vi "sonarPositionUpdate.vi"(1 "Obstacles":dbl[][](array[numeric]), 2 "Robot Properties In":T1={"Position"=[0.0, 0.0], "Size"=50.0, "Facing"=0.0, "Movement Ratios"=[0.0, -1.0], "Wheel Angle"=0.0}) -> (0 "Robot Properties Out":T1={"Position"=[0.0, 0.0], "Size"=50.0, "Facing"=0.0, "Movement Ratios"=[0.0, -1.0], "Wheel Angle"=0.0})   [LabVIEW 2015]
uses:
  Robot.ctl
  class/SonarSensor.lvclass
  class/Car.lvclass
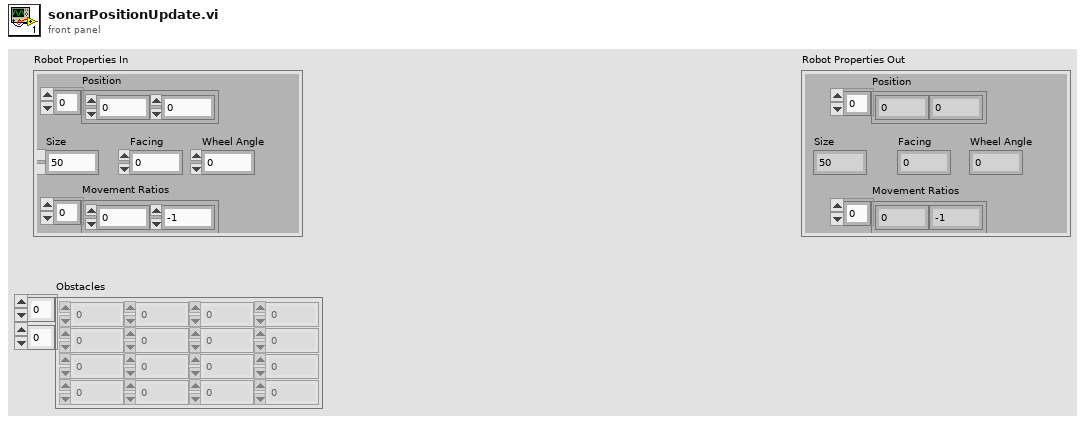
[diagram p1: front panel]
types:
  T1 = typedef "Robot.ctl" = cluster{"Position":dbl[], "Size":dbl, "Facing":dbl, "Movement Ratios":dbl[], "Wheel Angle":dbl}
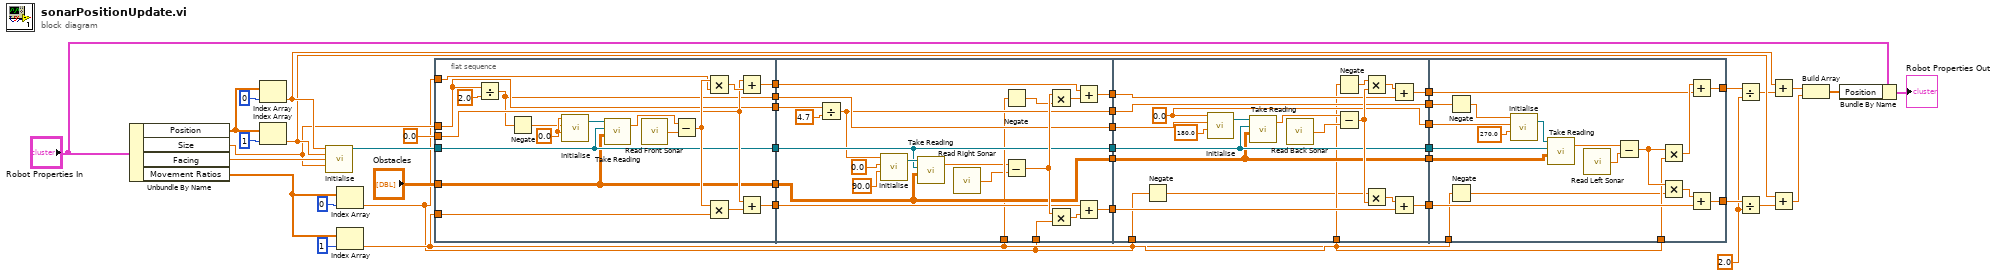
[diagram p0: block diagram]
diagram:
  w2 = 2.0 ("y")
  n1 = Unbundle By Name("Robot Properties In") -> ("Position"=w42:dbl[], "Size"=w24:dbl, "Facing"=w40:dbl, "Movement Ratios"=w37:dbl[])
  n2 = Index Array(array=w42, index=0) -> (element=w28:dbl)
  n3 = Index Array(array=w42, index=1) -> (element=w27:dbl)
  n4 = call "Initialise.vi"("X"=w28, "Y"=w27, "Facing"=w40, "Size"=w24) -> ("Car.lvclass"=w38:refnum<class "Car.lvclass">)  [unwired: 10 in, 1 out]
  n5 = Index Array(array=w37, index=0) -> (element=w6:dbl)
  n6 = Index Array(array=w37, index=1) -> (element=w7:dbl)
  n7 = flat-sequence {
    tunnel: w38 -> [w48]
    tunnel: "Obstacles" -> [w47]
    tunnel: w6 -> [w46]
    tunnel: w7 -> [w45]
    tunnel: 0.0 -> [w52]
    tunnel: [w54] -> w26
    tunnel: [w53] -> w25
    tunnel: w24 -> [w49]
    tunnel: [w49] -> w23
    tunnel: [w48] -> w22
    tunnel: [w47] -> w21
    tunnel: [w44] -> w17
    tunnel: w26 -> [w74]
    tunnel: w25 -> [w73]
    tunnel: w23 -> [w81]
    tunnel: w22 -> [w72]
    tunnel: w21 -> [w71]
    tunnel: [w72] -> w20
    tunnel: [w71] -> w19
    tunnel: [w70] -> w18
    tunnel: w17 -> [w70]
    tunnel: [w69] -> w16
    tunnel: [w68] -> w15
    tunnel: [w67] -> w11
    tunnel: w6 -> [w66]
    tunnel: w7 -> [w64]
    tunnel: w20 -> [w92]
    tunnel: w19 -> [w91]
    tunnel: w18 -> [w100]
    tunnel: w16 -> [w94]
    tunnel: w15 -> [w93]
    tunnel: [w92] -> w14
    tunnel: [w91] -> w13
    tunnel: [w90] -> w12
    tunnel: w11 -> [w89]
    tunnel: [w89] -> w10
    tunnel: [w87] -> w9
    tunnel: [w86] -> w8
    tunnel: w6 -> [w85]
    tunnel: w7 -> [w83]
    tunnel: w14 -> [w120]
    tunnel: w13 -> [w119]
    tunnel: w12 -> [w118]
    tunnel: w10 -> [w116]
    tunnel: w9 -> [w111]
    tunnel: w8 -> [w110]
    tunnel: [w109] -> w3
    tunnel: [w108] -> w4
    tunnel: w7 -> [w107]
    tunnel: w6 -> [w104]
    frame #0 {
      w61 = 0.0
      n8 = Divide(x=w49, y=2.0) -> (x/y=w44:dbl)
      n9 = Negate(x=w44) -> (-x=w50:dbl)
      n10 = call "Initialise.vi"("Facing"=w61, "Y"=w50, "X"=w61) -> ("SonarSensor.lvclass"=w60:refnum<class "SonarSensor.lvclass">)  [unwired: 1 in, 1 out]
      n11 = call "Take Reading.vi"("Obstacle Boundries"=w47, "Car.lvclass"=w48, "SonarSensor.lvclass"=w60) -> ("Distance Read"=w59:dbl)  [unwired: 1 in, 1 out]
      n12 = call "Read Front Sonar.vi"() -> ("Distance(cm)"=w58:dbl)  [unwired: 1 in]
      n13 = Subtract(x=w59, y=w58) -> (x-y=w57:dbl)
      n14 = Multiply(x=w57, y=w46) -> (x*y=w56:dbl)
      n15 = Multiply(x=w57, y=w45) -> (x*y=w55:dbl)
      n16 = Add(x=w52, y=w56) -> (x+y=w53:dbl)
      n17 = Add(x=w52, y=w55) -> (x+y=w54:dbl)
    }
    frame #1 {
      n18 = Divide(x=w81, y=4.7) -> (x/y=w67:dbl)
      n19 = call "Initialise.vi"("Facing"=90.0, "Y"=0.0, "X"=w67) -> ("SonarSensor.lvclass"=w78:refnum<class "SonarSensor.lvclass">)  [unwired: 1 in, 1 out]
      n20 = call "Take Reading.vi"("Obstacle Boundries"=w71, "Car.lvclass"=w72, "SonarSensor.lvclass"=w78) -> ("Distance Read"=w63:dbl)  [unwired: 1 in, 1 out]
      n21 = call "Read Right Sonar.vi"() -> ("Distance(cm)"=w62:dbl)  [unwired: 1 in]
      n22 = Negate(x=w64) -> (-x=w65:dbl)
      n23 = Subtract(x=w63, y=w62) -> (x-y=w77:dbl)
      n24 = Multiply(x=w77, y=w65) -> (x*y=w76:dbl)
      n25 = Multiply(x=w77, y=w66) -> (x*y=w75:dbl)
      n26 = Add(x=w73, y=w76) -> (x+y=w68:dbl)
      n27 = Add(x=w74, y=w75) -> (x+y=w69:dbl)
    }
    frame #2 {
      w90 = 0.0 ("X")
      n28 = Negate(x=w83) -> (-x=w84:dbl)
      n29 = call "Initialise.vi"("Facing"=180.0, "Y"=w100, "X"=w90) -> ("SonarSensor.lvclass"=w102:refnum<class "SonarSensor.lvclass">)  [unwired: 1 in, 1 out]
      n30 = call "Take Reading.vi"("Obstacle Boundries"=w91, "Car.lvclass"=w92, "SonarSensor.lvclass"=w102) -> ("Distance Read"=w99:dbl)  [unwired: 1 in, 1 out]
      n31 = call "Read Back Sonar.vi"() -> ("Distance(cm)"=w98:dbl)  [unwired: 1 in]
      n32 = Negate(x=w85) -> (-x=w88:dbl)
      n33 = Subtract(x=w99, y=w98) -> (x-y=w97:dbl)
      n34 = Multiply(x=w88, y=w97) -> (x*y=w96:dbl)
      n35 = Multiply(x=w84, y=w97) -> (x*y=w95:dbl)
      n36 = Add(x=w96, y=w93) -> (x+y=w87:dbl)
      n37 = Add(x=w95, y=w94) -> (x+y=w86:dbl)
    }
    frame #3 {
      n38 = Negate(x=w116) -> (-x=w117:dbl)
      n39 = Negate(x=w107) -> (-x=w103:dbl)
      n40 = call "Initialise.vi"("Facing"=270.0, "Y"=w118, "X"=w117) -> ("SonarSensor.lvclass"=w121:refnum<class "SonarSensor.lvclass">)  [unwired: 1 in, 1 out]
      n41 = call "Take Reading.vi"("Obstacle Boundries"=w119, "Car.lvclass"=w120, "SonarSensor.lvclass"=w121) -> ("Distance Read"=w106:dbl)  [unwired: 1 in, 1 out]
      n42 = call "Read Left Sonar.vi"() -> ("Distance(cm)"=w105:dbl)  [unwired: 1 in]
      n43 = Subtract(x=w106, y=w105) -> (x-y=w114:dbl)
      n44 = Multiply(x=w114, y=w104) -> (x*y=w113:dbl)
      n45 = Multiply(x=w114, y=w103) -> (x*y=w112:dbl)
      n46 = Add(x=w113, y=w111) -> (x+y=w109:dbl)
      n47 = Add(x=w112, y=w110) -> (x+y=w108:dbl)
    }
  }
  n48 = Divide(x=w3, y=w2) -> (x/y=w1:dbl)
  n49 = Divide(x=w4, y=w2) -> (x/y=w5:dbl)
  n50 = Add(x=w28, y=w1) -> (x+y=w30:dbl)
  n51 = Add(x=w27, y=w5) -> (x+y=w29:dbl)
  n52 = Build Array(w30, w29) -> (w31:dbl[])
  n53 = Bundle By Name(cluster="Robot Properties In", "Position"=w31) -> (→"Robot Properties Out":T1)
